vi "OBJ_SetS.vi"(2 "value index IN":i32, 3 "value IN":string, 4 "object handle IN":i32) -> (0 "error code OUT":i32, 1 "object handle OUT":i32)   [LabVIEW 2016]
doc: "Sets a properties value from a string.\n\nThis is a property related function and it will fail if this object does not\nreference a property.\n\nEyery properties value can be set as from a string.\n\nIf this property stores more then one value the 'value index IN' terminal can be used to specify which value to query.\n\nThe 'error code OUT' terminal will deliver 0 if successful or a negative error code otherwise. A list of valid error codes and their meaning can be found in the manual about this interface."
uses:
  mvDeviceManager.dll
panel:
  # "INPUT"
  # "OUTPUT"
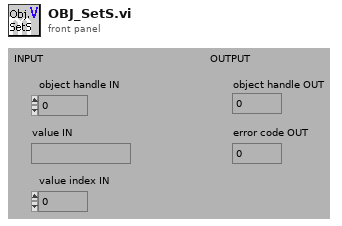
[diagram p1: front panel]
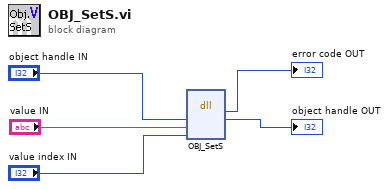
[diagram p0: block diagram]
diagram:
  n1 = dll-call lib="mvDeviceManager.dll" fn="OBJ_SetS"("hObj"="object handle IN", "value"="value IN", "index"="value index IN") -> (→"error code OUT":i32, "hObj"=→"object handle OUT":i32)  [unwired: 5 in, 2 out]
